vi "APX VarianTMP HEM.vi"() -> ()   [LabVIEW 2015]
uses:
  <vilib>/Instr/_visa.llb/VISA Configure Serial Port (Instr).vi
  <userlib>/caLab/Private/Get_PV-1D.vi
  <userlib>/caLab/Private/Put_DBL-1D_PV-1D.vi
  <userlib>/caLab/Private/Put_DBL_PV.vi
panel:
  out "APX:HEMTurboS":dbl
  out "TMPC5STRSTP 2":string
  out "APX:HEMTurbo_STOP":bool
  out "APX:HEMTurbo_START":bool
  out "TMPC5STRSTP":string
  out "SERIAL":string
  out "V-304":refnum<visa-resource-name>="COM4"
  out "APX:HEMTurboF":dbl caption="F_20/Hz"
  out "APX:HEMTurboP":dbl caption="P_20/W"
  out "APX:HEMTurboS:STR":string
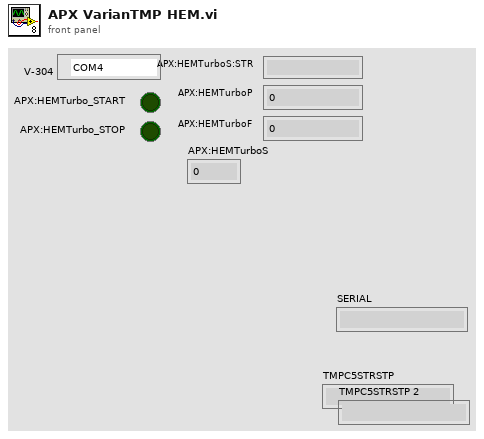
[diagram p1: front panel]
types:
  T1 = enum16{"START", "STOP", "REMOTE/SERIAL", "REMOTE", "SERIAL", "START/STOP", "PUMP STATUS", "Driving Frequency", "PUMP POWER", "PRESSURE"}
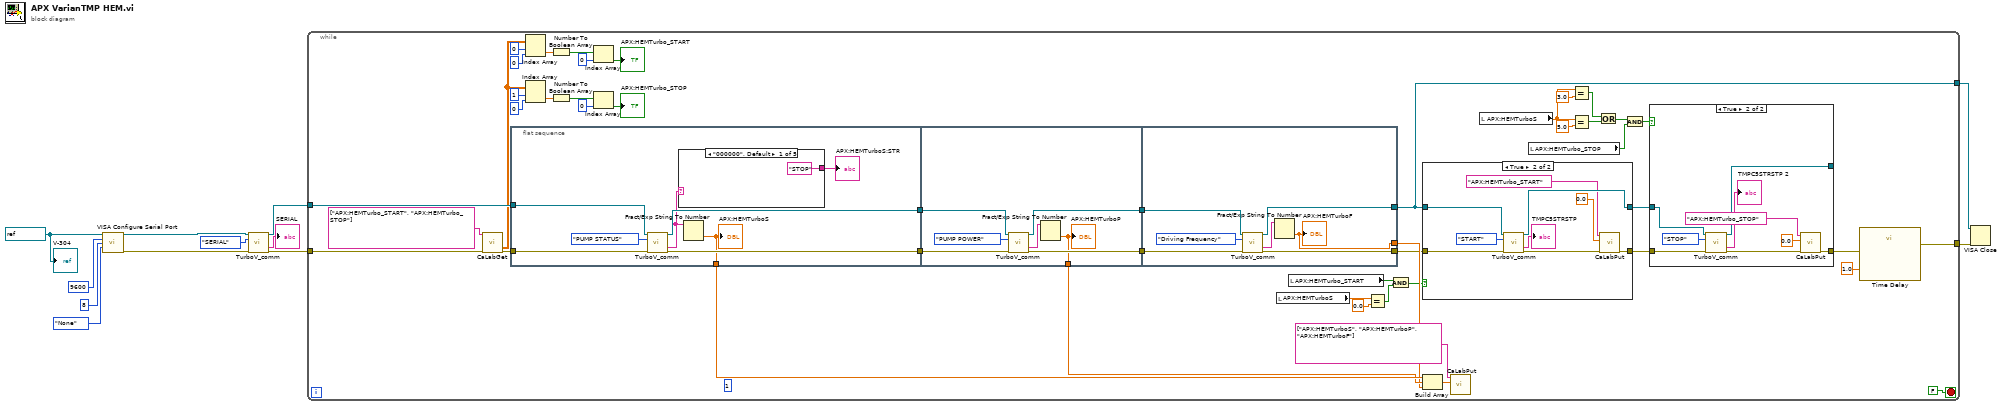
[diagram p0: block diagram]
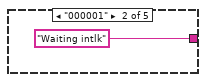
[diagram p2: hidden frame]
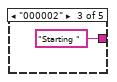
[diagram p3: hidden frame]
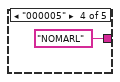
[diagram p4: hidden frame]
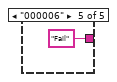
[diagram p5: hidden frame]
diagram:
  w12 = refnum<visa-resource-name> "COM5" ("VISA resource name")
  n1 = call-poly "VISA Configure Serial Port"("VISA resource name"=w12, "baud rate (9600)"=u32 9600, "data bits (8)"=u16 8, "parity (0:none)"=enum16{"None", "Odd", "Even", "Mark", "Space"}."None") -> ("VISA resource name out"=w5:refnum<visa-resource-name>, "error out"=w3:errorcluster)  [unwired: 10 in]
  n2 = call "TurboV_comm.vi"("VISA resource name"=w5, "Command"=T1."SERIAL", "error in (no error)"=w3) -> ("VISA resource name out"=w4:refnum<visa-resource-name>, "read buffer"=→"SERIAL":string, "error out"=w2:errorcluster)  [unwired: 10 in]
  n3 = while {
    tunnel: w4 -> [w59]
    tunnel: w2 -> [w39]
    tunnel: [w23] -> w8
    tunnel: [w57] -> w7
    stop <- FALSE stop-if-true
    (unwired) 1
    n4 = call-poly "CaLabGet.vi"("PV Names"=string[] ["APX:HEMTurbo_START", "APX:HEMTurbo_STOP"], "Error in (no error)"=w39) -> ("Value Array (number)"=w40:dbl[][], "Error out"=w38:errorcluster)  [unwired: 7 in, 5 out]
    n5 = flat-sequence {
      tunnel: w59 -> [w67]
      tunnel: w38 -> [w66]
      tunnel: [w65] -> w28
      tunnel: [w64] -> w27
      tunnel: [w60] -> w55
      tunnel: w28 -> [w78]
      tunnel: w27 -> [w75]
      tunnel: [w77] -> w26
      tunnel: [w76] -> w25
      tunnel: [w73] -> w54
      tunnel: w26 -> [w86]
      tunnel: w25 -> [w85]
      tunnel: [w82] -> w22
      tunnel: [w81] -> w23
      tunnel: [w80] -> w53
      frame #0 {
        n6 = call "TurboV_comm.vi"("VISA resource name"=w67, "Command"=T1."PUMP STATUS", "error in (no error)"=w66) -> ("VISA resource name out"=w65:refnum<visa-resource-name>, "read buffer"=w61:string, "error out"=w64:errorcluster)  [unwired: 10 in]
        n7 = case shown="\"000000\", Default" w61 {
          tunnel: ["STOP" "Waiting intlk" "Starting " "NOMARL" "Fail"] -> w62
          frame "000000", Default {
          }
          frame "000001" {
          }
          frame "000002" {
          }
          frame "000005" {
          }
          frame "000006" {
          }
        }
        "APX:HEMTurboS:STR" <- w62
        n8 = Fract/Exp String To Number(string=w61) -> (number=w60:dbl)  [unwired: 3 in, 1 out]
        "APX:HEMTurboS" <- w60
      }
      frame #1 {
        n9 = call "TurboV_comm.vi"("VISA resource name"=w78, "Command"=T1."PUMP POWER", "error in (no error)"=w75) -> ("VISA resource name out"=w77:refnum<visa-resource-name>, "read buffer"=w74:string, "error out"=w76:errorcluster)  [unwired: 10 in]
        n10 = Fract/Exp String To Number(string=w74) -> (number=w73:dbl)  [unwired: 3 in, 1 out]
        "APX:HEMTurboP" <- w73
      }
      frame #2 {
        n11 = call "TurboV_comm.vi"("VISA resource name"=w86, "Command"=T1."Driving Frequency", "error in (no error)"=w85) -> ("VISA resource name out"=w81:refnum<visa-resource-name>, "read buffer"=w83:string, "error out"=w82:errorcluster)  [unwired: 10 in]
        n12 = Fract/Exp String To Number(string=w83) -> (number=w80:dbl)  [unwired: 3 in, 1 out]
        "APX:HEMTurboF" <- w80
      }
    }
    n13 = Index Array(array=w40, index (row)=0 ("disabled index (row)"), index (col)=0 ("index (row)")) -> (element=w46:dbl)
    n14 = Index Array(array=w40, index (row)=1 ("disabled index (row)"), index (col)=0 ("index (row)")) -> (element=w41:dbl)
    n15 = Number To Boolean Array(number=w46) -> (Boolean array=w48:bool[])
    n16 = Number To Boolean Array(number=w41) -> (Boolean array=w43:bool[])
    n17 = Index Array(array=w48, index=0) -> (element=→"APX:HEMTurbo_START":bool)
    n18 = Index Array(array=w43, index=0) -> (element=→"APX:HEMTurbo_STOP":bool)
    n19 = local read "APX:HEMTurboS"() -> (w29:dbl)
    n20 = local read "APX:HEMTurbo_START"() -> (w18:bool)
    n21 = Equal?(x=w29, y=0.0) -> (x = y?=w17:bool)
    n22 = And(x=w18, y=w17) -> (x .and. y?=w16:bool)
    n23 = case shown="True" w16 {
      tunnel: [w88 w95] -> w21
      tunnel: [w87 w89] -> w20
      tunnel: w23 -> [w88 w94]
      tunnel: w22 -> [w87 w93]
      frame False {
      }
      frame True {
        n24 = call "TurboV_comm.vi"("VISA resource name"=w94, "Command"=T1."START", "error in (no error)"=w93) -> ("VISA resource name out"=w95:refnum<visa-resource-name>, "read buffer"=→"TMPC5STRSTP":string, "error out"=w90:errorcluster)  [unwired: 10 in]
        n25 = call-poly <userlib>:"CaLabPut.vi"("Error in (no error)"=w90, "Value"=0.0, "PV Name"="APX:HEMTurbo_START") -> ("Error out"=w89:errorcluster)  [unwired: 5 in, 3 out]
      }
    }
    n26 = Build Array(w55, w54, w53) -> (w52:dbl[])
    n27 = call-poly <userlib>:"CaLabPut.vi"("Values"=w52, "PV Names"=string[] ["APX:HEMTurboS", "APX:HEMTurboP", "APX:HEMTurboF"]) -> ()  [unwired: 6 in, 4 out]
    n28 = local read "APX:HEMTurboS"() -> (w35:dbl)
    n29 = local read "APX:HEMTurbo_STOP"() -> (w13:bool)
    n30 = Equal?(x=w35, y=3.0) -> (x = y?=w33:bool)
    n31 = Equal?(x=w35, y=5.0) -> (x = y?=w34:bool)
    n32 = Or(x=w33, y=w34) -> (x .or. y?=w15:bool)
    n33 = And(x=w15, y=w13) -> (x .and. y?=w14:bool)
    n34 = case shown="True" w14 {
      tunnel: w21 -> [w99 w107]
      tunnel: w20 -> [w98 w106]
      tunnel: [w99 w102] -> _
      tunnel: [w98 w100] -> w19
      frame False {
      }
      frame True {
        n35 = call "TurboV_comm.vi"("VISA resource name"=w107, "Command"=T1."STOP", "error in (no error)"=w106) -> ("VISA resource name out"=w102:refnum<visa-resource-name>, "read buffer"=→"TMPC5STRSTP 2":string, "error out"=w101:errorcluster)  [unwired: 10 in]
        n36 = call-poly <userlib>:"CaLabPut.vi"("Error in (no error)"=w101, "Value"=0.0, "PV Name"="APX:HEMTurbo_STOP") -> ("Error out"=w100:errorcluster)  [unwired: 5 in, 3 out]
      }
    }
    n37 = call "Time Delay"("error in (no error)"=w19, "Delay Time (s)"=1.0) -> ("error out"=w57:errorcluster)  [unwired: 9 in]
  }
  n38 = VISA Close(VISA resource name=w8, error in (no error)=w7) -> ()  [unwired: 1 out]
  "V-304" <- w12
